vi "CRYGet Window Menu.vi"(10 "Tags":string[](array[string])=["VIEW_STEP_SETUP", "VIEW_DATA_VIEW", "VIEW_DOCUMENT", "TOOLS_PAUSE", "TOOLS_START", "TOOLS_STOP", "TOOLS_CONTINUE", "OPERATOR_SIGGEN", "OPERATOR_MULTIMETER", "OPERATOR_OSCILLOSCOPE", "OPERATOR_SPECTRUM", "OPERATOR_RTA", "VIEW_PROJECT", "VIEW_CURVES_LIBRARY"]) -> (0 "NamesTF_Out":bool[](array[boolean]), 1 "Tags_Out":string[](array[string])=["VIEW_STEP_SETUP", "VIEW_DATA_VIEW", "VIEW_PROJECT_DOCUMENT", "TOOLS_PAUSE", "TOOLS_START", "TOOLS_STOP", "TOOLS_Continue", "OPERATOR_SIGGEN", "OPERATOR_MULTIMETER", "OPERATOR_OSCILLOSCOPE", "OPERATOR_SPECTRUM", "OPERATOR_RTA", "VIEW_PROJECT", "VIEW_CURVES_LIBRARY"], 2 "Names_Out":string[](array[string])=["Step Setup", "Data View", "Document", "Pause", "Start", "Stop", "Continue", "Signal Generator", "Multimeter", "Oscilloscope", "Spectrum _Analyzer", "RealTime Analyzer", "_Project", "_Curves Library"])   [LabVIEW 2013]
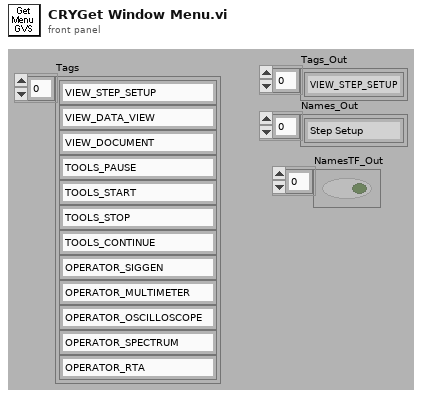
[diagram p1: front panel]
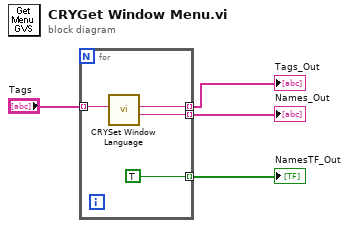
[diagram p0: block diagram]
diagram:
  n1 = for {
    tunnel: "Tags" -> [w8] mode=indexing
    tunnel: [w7] -> w2 mode=indexing
    tunnel: [w6] -> w1 mode=indexing
    tunnel: [TRUE] -> w4 mode=indexing
    n2 = call "CRYSet Window Language.vi"("sID"=w8) -> ("sMultibyte_Out"=w6:string, "sID_Out"=w7:string)  [unwired: 8 in, 1 out]
  }
  "Tags_Out" <- w2
  "Names_Out" <- w1
  "NamesTF_Out" <- w4
